vi "DSKNM.vi"(11 "file path":path) -> (0 "tmpArr":string[][](array[string]), 1 "Money":dbl[](array[numeric]), 3 "TableRes":string[][](table))   [LabVIEW 2023]
uses:
  DskTypeDef.ctl
panel:
  in  "stop":bool
  out "min index":i32
  out "minDate":string[](array[string])
  out "maxDate":string[](array[string])
  out "Min":dbl format="%#_5g"
  out "Max":dbl format="%#_6f"
  out "All Sum":dbl
  out "Transfer numbers":i32
  out "Waveform Chart":i32(graph)
  in  "Transaction Type":T1
  # "$"
  # "$"
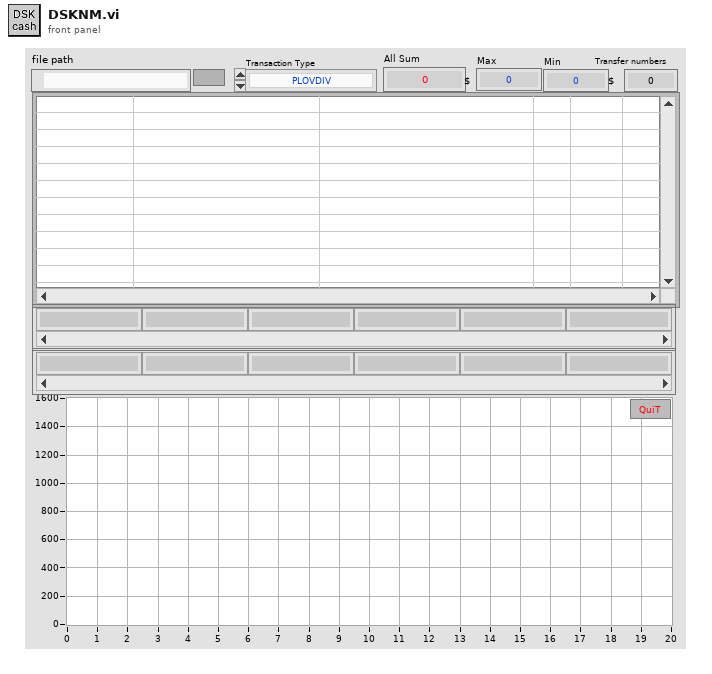
[diagram p1: front panel]
types:
  T1 = typedef "DskTypeDef.ctl" = enum16{"PLOVDIV", "ПЛАЩАНЕ НА ПОС", "RAKOVSKI", "VRATSA", "KOZLODUI", "SOFIA", "MOTARS", "SMS/VIBER", "ТАКСА ПАКЕТНО ОБСЛУЖВАНЕ", "ЛИХВА", "СБКО", "ТЕГЛЕНЕ", "ЗАЕМ", "BREZOVO", "VIVACOM", "ЕЛЕКТРОХОЛД", "ЕВН", "ЗАПЛАТА", "АВАНС", "НЕТ", "ТРАНСФЕР"}
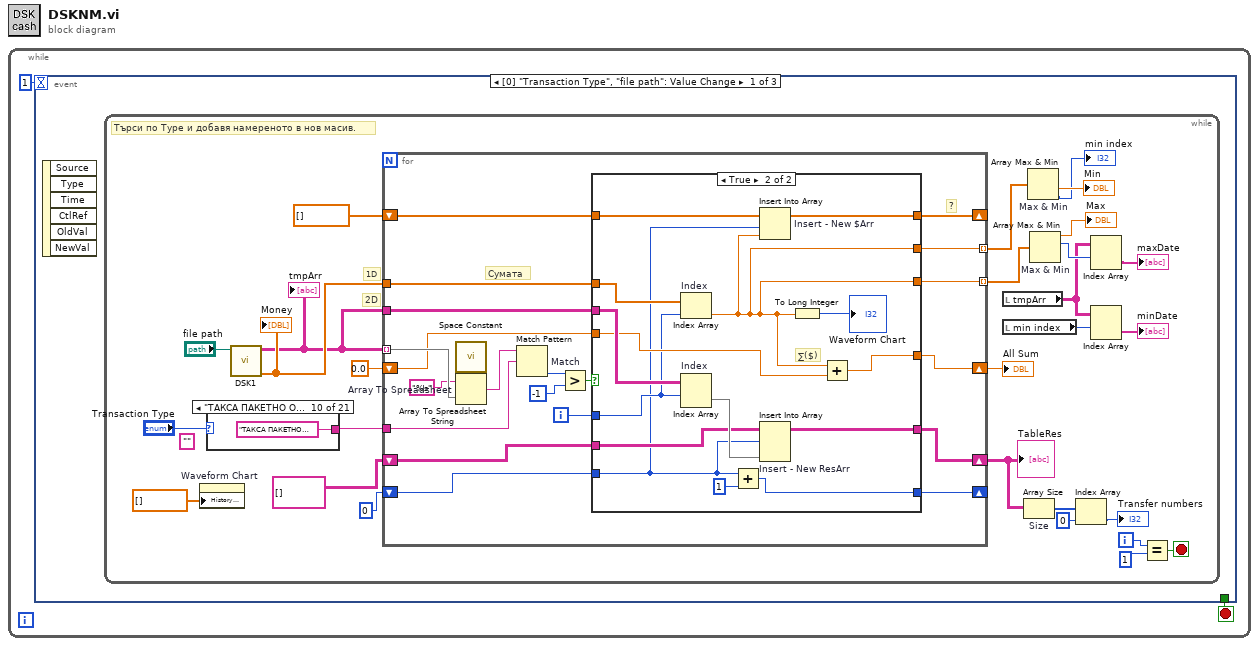
[diagram p0: block diagram]
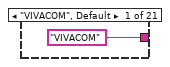
[diagram p2: hidden frame]
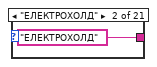
[diagram p3: hidden frame]
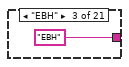
[diagram p4: hidden frame]
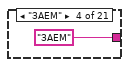
[diagram p5: hidden frame]
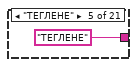
[diagram p6: hidden frame]
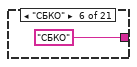
[diagram p7: hidden frame]
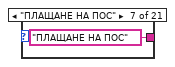
[diagram p8: hidden frame]
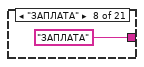
[diagram p9: hidden frame]
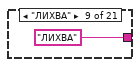
[diagram p10: hidden frame]
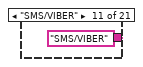
[diagram p11: hidden frame]
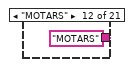
[diagram p12: hidden frame]
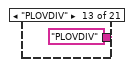
[diagram p13: hidden frame]
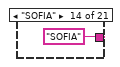
[diagram p14: hidden frame]
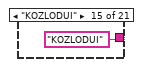
[diagram p15: hidden frame]
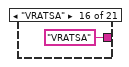
[diagram p16: hidden frame]
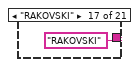
[diagram p17: hidden frame]
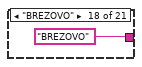
[diagram p18: hidden frame]
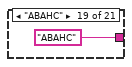
[diagram p19: hidden frame]
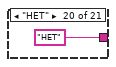
[diagram p20: hidden frame]
diagram:
  n1 = while {
    stop <- w2 stop-if-true
    n2 = event shown="[0] \"Transaction Type\", \"file path\": Value Change" {
      selector: _ -> [_ _ _]
      dyn-events: _ -> [_ _ _]
      timeout: 1 -> [_ _ _]
      tunnel: [_ "stop" _] -> w2
      event "file path": Value Change {
        n3 = event-data() -> ()  [unwired: 1 in, 6 out]
        n4 = while {
          i -> [w8]
          stop <- w6 stop-if-true
          (unwired) ""
          # "Търси по Type и добавя намереното в нов масив."
          # "2D"
          # "1D"
          n5 = property on="Waveform Chart" class="WFChart (strict)"("History Data"=dbl[] []) -> ()  [unwired: 2 in, 2 out]
          n6 = case shown="\"ТАКСА ПАКЕТНО ОБСЛУЖВАНЕ\"" "Transaction Type" {
            tunnel: ["VIVACOM" "ЕЛЕКТРОХОЛД" "ЕВН" "ЗАЕМ" "ТЕГЛЕНЕ" "СБКО" "ПЛАЩАНЕ НА ПОС" "ЗАПЛАТА" "ЛИХВА" "ТАКСА ПАКЕТНО ОБСЛУЖВАНЕ" "SMS/VIBER" "MOTARS" "PLOVDIV" "SOFIA" "KOZLODUI" "VRATSA" "RAKOVSKI" "BREZOVO" "АВАНС" "НЕТ" "ТРАНСФЕР"] -> w28
            frame "VIVACOM", Default {
            }
            frame "ЕЛЕКТРОХОЛД" {
            }
            frame "ЕВН" {
            }
            frame "ЗАЕМ" {
            }
            frame "ТЕГЛЕНЕ" {
            }
            frame "СБКО" {
            }
            frame "ПЛАЩАНЕ НА ПОС" {
            }
            frame "ЗАПЛАТА" {
            }
            frame "ЛИХВА" {
            }
            frame "ТАКСА ПАКЕТНО ОБСЛУЖВАНЕ" {
            }
            frame "SMS/VIBER" {
            }
            frame "MOTARS" {
            }
            frame "PLOVDIV" {
            }
            frame "SOFIA" {
            }
            frame "KOZLODUI" {
            }
            frame "VRATSA" {
            }
            frame "RAKOVSKI" {
            }
            frame "BREZOVO" {
            }
            frame "АВАНС" {
            }
            frame "НЕТ" {
            }
            frame "ТРАНСФЕР" {
            }
          }
          n7 = call "DSK1.vi"("file path (dialog if empty)"="file path") -> ("Money"=w4:dbl[], "Transfers"=w3:string[][])  [unwired: 6 in, 3 out]
          "tmpArr" <- w3
          "Money" <- w4
          n8 = for {
            tunnel: w3 -> [w64] mode=indexing
            tunnel: w28 -> [w65]
            tunnel: w3 -> [w71]
            shift-right: [w68] -> _
            shift-left: 0 -> [w69]
            shift-right: [w67] -> w24
            shift-left: string[][] [] -> [w66]
            tunnel: w4 -> [w58]
            shift-right: [w56] -> w20
            shift-left: 0.0 -> [w57]
            shift-right: [w55] -> _
            shift-left: dbl[] [] -> [w54]
            tunnel: [w53] -> w16 mode=indexing
            tunnel: [w52] -> w12 mode=indexing
            i -> [w70]
            # "?"
            # "Сумата"
            n9 = call <vilib>:"Space Constant.vi"() -> ("String"=w63:string)
            n10 = Array To Spreadsheet String "Array To Spreadsheet"(delimiter (Tab)=w63, array=w64, 3:"%s" ("format string")) -> (spreadsheet string=w62:string)
            n11 = Match Pattern "Match"(string=w62, regular expression=w65) -> (offset past match=w59:i32)  [unwired: 1 in, 3 out]
            n12 = Greater?(x=w59, y=-1) -> (0:w72:bool)
            n13 = case shown="True" w72 {
              tunnel: w71 -> [_ w92]
              tunnel: w70 -> [_ w83]
              tunnel: w69 -> [w76 w80]
              tunnel: [w76 w90] -> w68
              tunnel: [w77 w89] -> w67
              tunnel: w66 -> [w77 w87]
              tunnel: w58 -> [_ w84]
              tunnel: [w75 w86] -> w56
              tunnel: w57 -> [w75 w85]
              tunnel: [w74 w82] -> w55
              tunnel: w54 -> [w74 w81]
              tunnel: [_ w79] -> w53
              tunnel: [1000000000000.0 w79] -> w52
              frame False {
                # "Трябваше ми нещо голямо ;)"
              }
              frame True {
                # "∑($)"
                n14 = Index Array "Index"(array=w84, index=w83) -> (element=w79:dbl)
                n15 = Index Array "Index"(array=w92, index (row)=w83) -> (element=w88:string[])  [unwired: 1 in]
                n16 = Add(x=w80, y=1) -> (x+y=w90:i32)
                n17 = Insert Into Array "Insert - New $Arr"(array=w81, index=w80, new element=w79) -> (w82:dbl[])
                n18 = Insert Into Array "Insert - New ResArr"(array=w87, index (row)=w80, new element=w88) -> (w89:string[][])  [unwired: 1 in]
                n19 = To Long Integer(number=w79) -> (32bit integer=→"Waveform Chart":i32)
                n20 = Add(x=w79, y=w85) -> (x+y=w86:dbl)
              }
            }
          }
          "All Sum" <- w20
          "TableRes" <- w24
          n21 = local read "tmpArr"() -> (w5:string[][])
          n22 = local read "min index"() -> (w9:i32)
          n23 = Array Size "Size"(array=w24) -> (size(s)=w23:i32[])
          n24 = Array Max & Min "Max & Min"(array=w12) -> (min value=→"Min":dbl, min index (indices)=→"min index":i32)  [unwired: 2 out]
          n25 = Array Max & Min "Max & Min"(array=w16) -> (max value=→"Max":dbl, max index (indices)=w15:i32)  [unwired: 2 out]
          n26 = Index Array(array=w23, index=0) -> (element=→"Transfer numbers":i32)
          n27 = Index Array(array=w5, index (row)=w15) -> (element=→"maxDate":string[])  [unwired: 1 in]
          n28 = Index Array(array=w5, index (row)=w9) -> (element=→"minDate":string[])  [unwired: 1 in]
          n29 = Equal?(x=w8, y=1) -> (x = y?=w6:bool)
        }
      }
      event "stop": Value Change {
        n30 = event-data() -> ()  [unwired: 1 in, 6 out]
        n31 = Quit LabVIEW(quit? (T)="stop") -> ()
      }
      event Timeout {
        n32 = event-data() -> ()  [unwired: 1 in, 3 out]
      }
    }
  }
